vi "programa 5.vi"() -> ()   [LabVIEW 2011]
uses:
  Control arreglo.ctl
panel:
  out "Array 2":bool[](array[boolean])
  out "Array":i32[](array[slide]) scale=0.0..60.0
  # "Encender un led cuando la temp sobrepase los 40 grados."
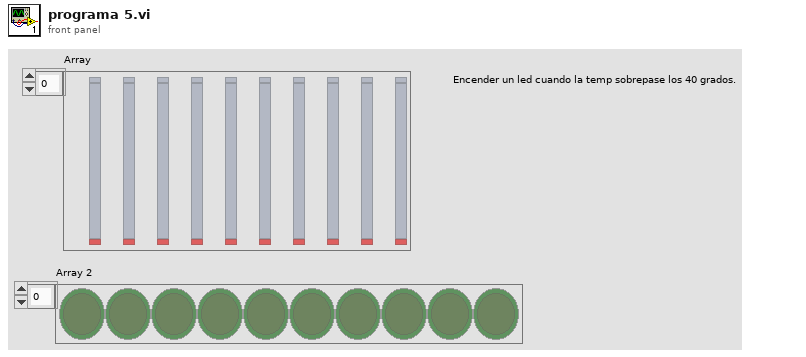
[diagram p1: front panel]
types:
  T1 = typedef "Control arreglo.ctl" = enum16{"Inicializar", "Rellenar Temp", "Encender led", "Final"}
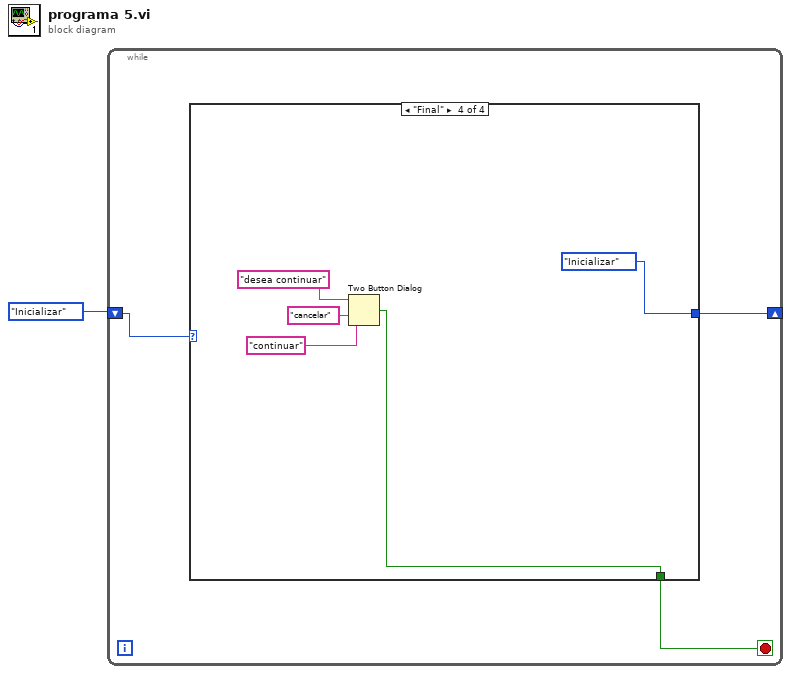
[diagram p0: block diagram]
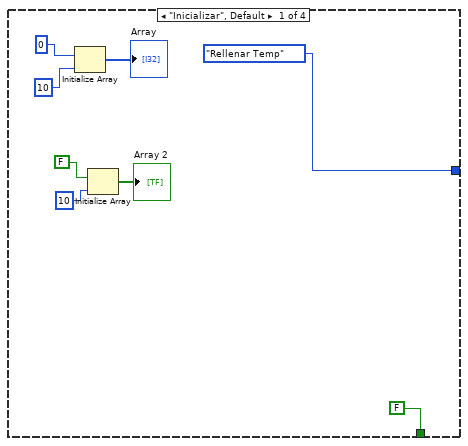
[diagram p2: hidden frame]
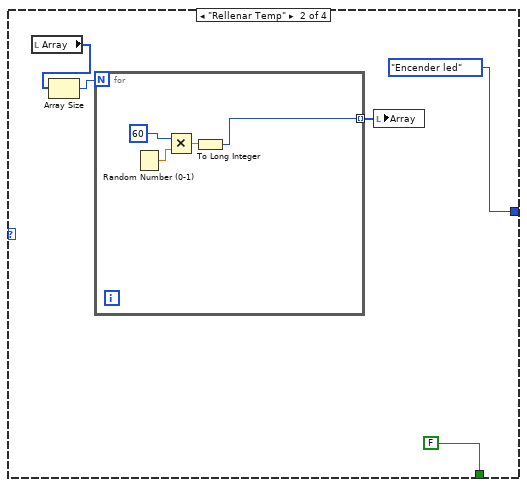
[diagram p3: hidden frame]
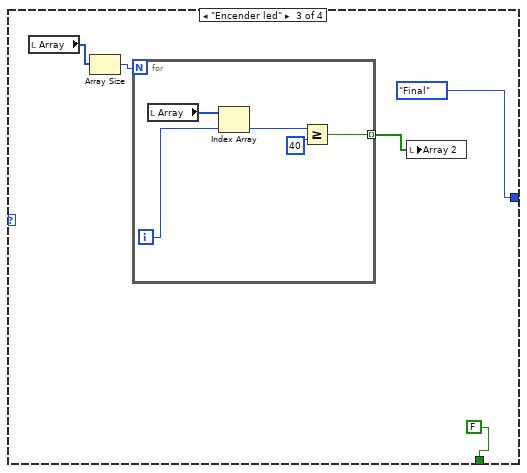
[diagram p4: hidden frame]
diagram:
  n1 = while {
    shift-right: [w3] -> _
    shift-left: Control_arreglo."Inicializar" -> [w4]
    stop <- w2 stop-if-true
    n2 = case shown="\"Final\"" w4 {
      tunnel: [Control_arreglo."Rellenar Temp" Control_arreglo."Encender led" Control_arreglo."Final" Control_arreglo."Inicializar"] -> w3
      tunnel: [FALSE FALSE FALSE w32] -> w2
      frame "Inicializar", Default {
        n3 = Initialize Array(0, 10) -> (→"Array":i32[])
        n4 = Initialize Array(FALSE, 10) -> (→"Array 2":bool[])
      }
      frame "Rellenar Temp" {
        n5 = local read "Array"() -> (w16:i32[])
        n6 = Array Size(array=w16) -> (size(s)=w17:i32)
        n7 = for {
          N: w17 -> [_]
          tunnel: [w18] -> w15 mode=indexing
          n8 = Random Number (0-1)() -> (number: 0 to 1=w19:dbl)
          n9 = Multiply(x=60, y=w19) -> (x*y=w21:dbl)
          n10 = To Long Integer(number=w21) -> (32bit integer=w18:i32)
        }
        n11 = local write "Array"(w15) -> ()
      }
      frame "Encender led" {
        n12 = local read "Array"() -> (w25:i32[])
        n13 = Array Size(array=w25) -> (size(s)=w26:i32)
        n14 = for {
          N: w26 -> [_]
          tunnel: [w27] -> w24 mode=indexing
          i -> [w30]
          n15 = local read "Array"() -> (w31:i32[])
          n16 = Index Array "Index Array"(array=w31, index=w30) -> (element=w29:i32)
          n17 = Greater Or Equal?(x=w29, y=40) -> (x >= y?=w27:bool)
        }
        n18 = local write "Array 2"(w24) -> ()
      }
      frame "Final" {
        n19 = Two Button Dialog(message="desea continuar", 1:"continuar" ("F button name (\"Cancel\")"), 2:"cancelar" ("T button name (\"OK\")")) -> (T button?=w32:bool)
      }
    }
  }
